vi "Update Trajectory.vi"(5 "Current Surgical Stage":T1(ring), 7 "Pattern":T2(ring)=enum."Centered", 8 "Depth Ctrl Array\n(% Thickness)":dbl[](array[numeric])=[40.0, 60.0, 80.0] min=10.0 max=90.0 step=5.0 format="%#_g%%", 9 "Scale":dbl=0.5, 10 "Offset":dbl[](array[numeric]), 11 "SCAN_NO":string="0011") -> (0 "Trajectory OOB":bool)   [LabVIEW 2016]
uses:
  Subsystems/Global Variables.vi
panel:
  in  "joint limits 1":dbl[][](array[numeric])=[[-8.0, 50.0], [-35.0, 35.0], [-5.0, 20.0], [-180.0, 180.0]] format="%#.3g"
  in  "Total Time":dbl=20.0
  in  "joint limits":dbl[][](array[numeric])=[[-68.0, -4.0], [-35.0, 35.0], [0.1, 10.0], [-40.0, 40.0]]
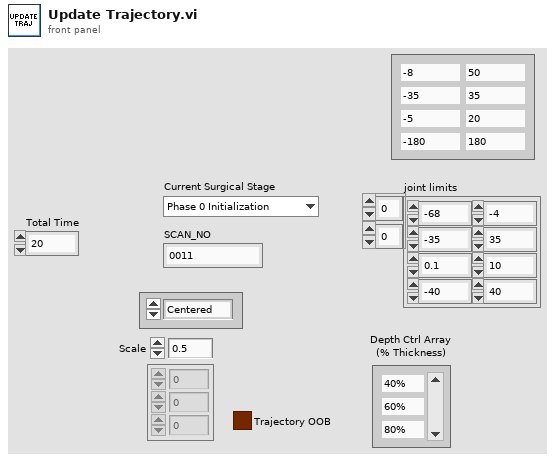
[diagram p1: front panel]
types:
  T1 = enum16{"Phase 0 Initialization", "Phase 1 Phaco", "Phase 2 Lens Removal", "Phase 3 IOL Injection"}
  T2 = enum16{"Entry Site", "Centered", "Insertion", "Extraction", "Reverse Entry Site", "Reverse Centered"}
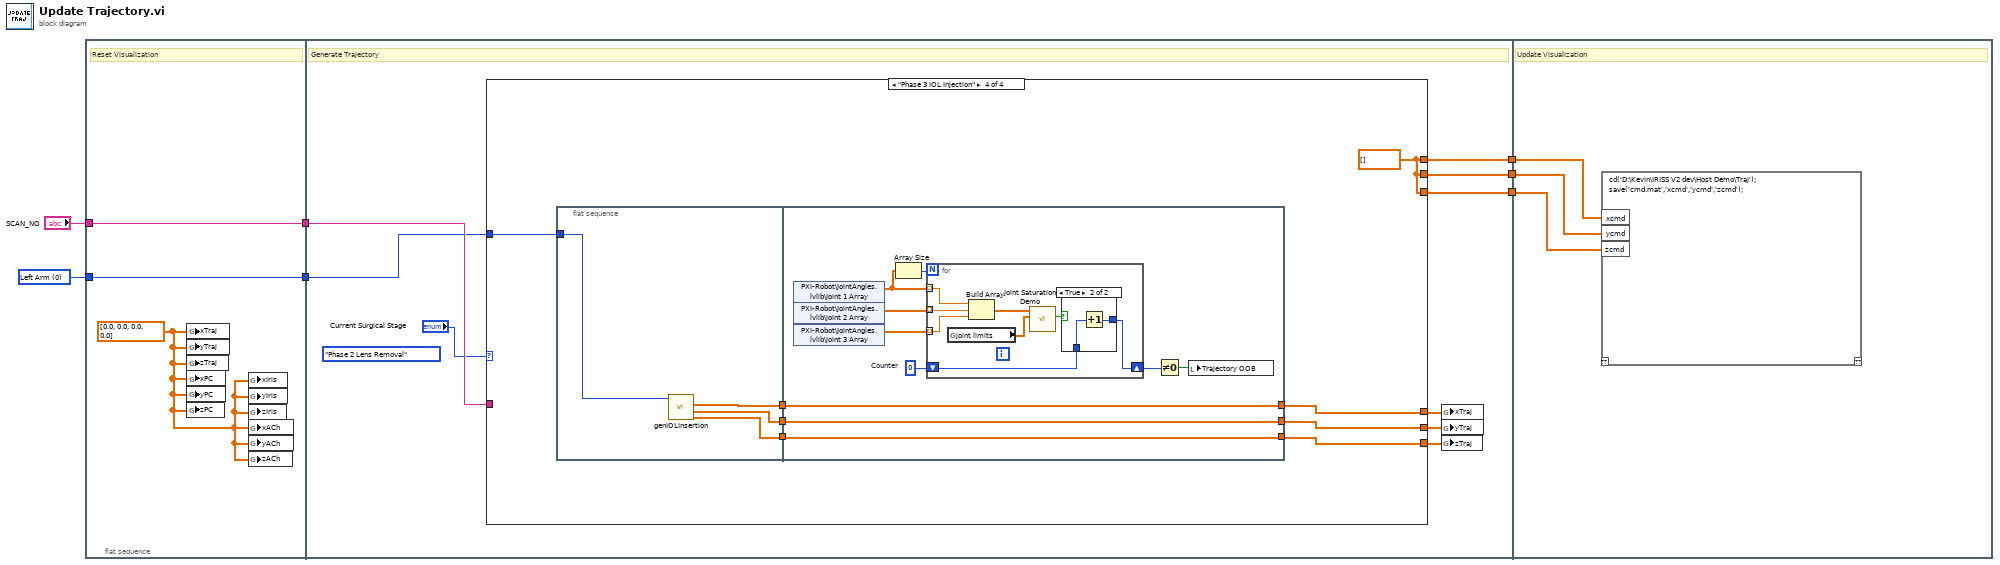
[diagram p0: block diagram]
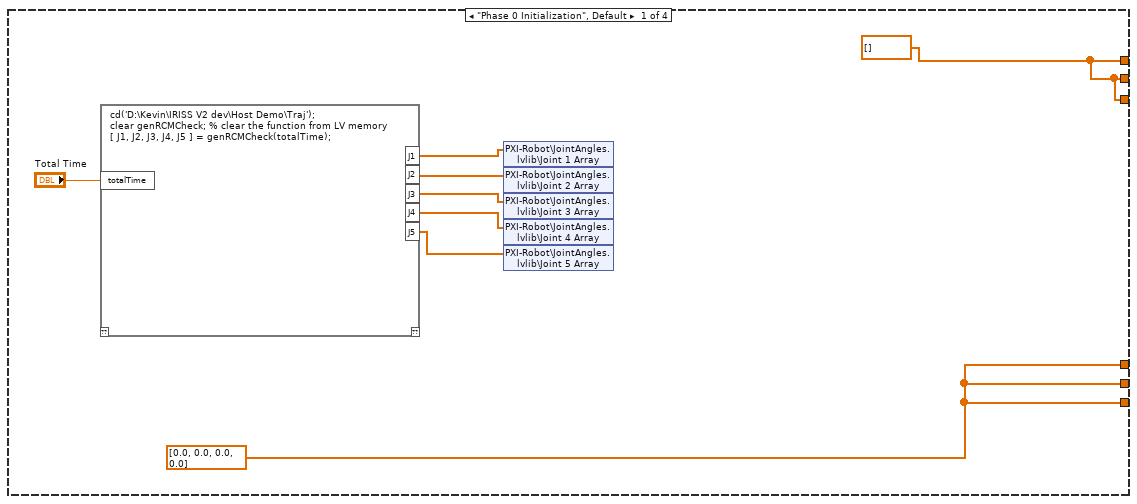
[diagram p2: hidden frame]
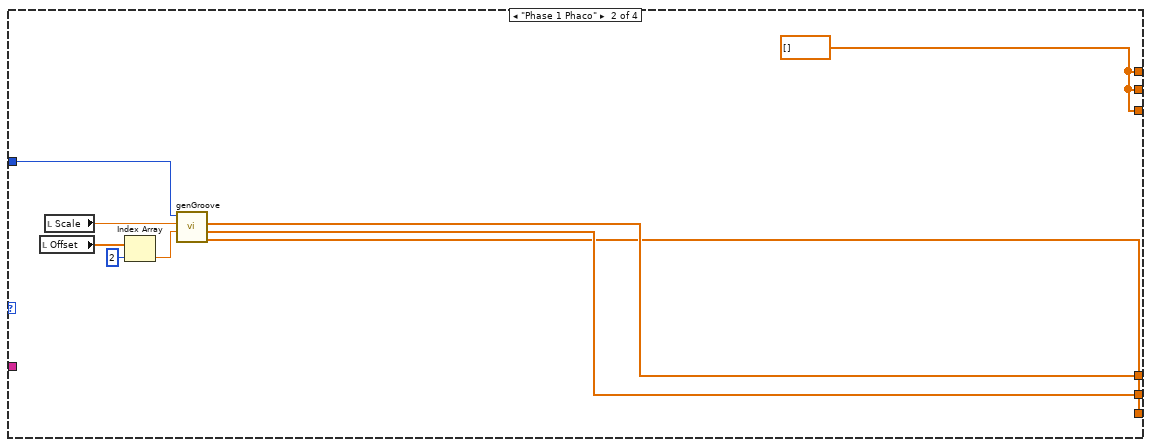
[diagram p3: hidden frame]
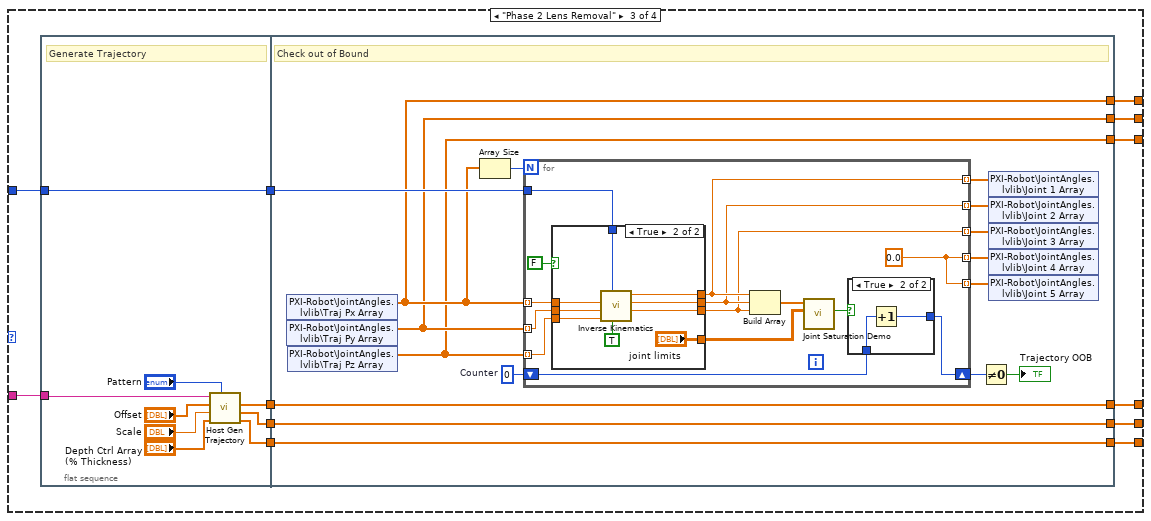
[diagram p4: hidden frame]
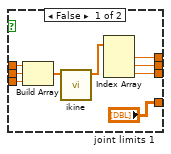
[diagram p5: hidden frame]
diagram:
  w4 = 0 items=["Left Arm", "Right Arm"] ("armID")
  n1 = flat-sequence {
    tunnel: "SCAN_NO" -> [w10]
    tunnel: [w10] -> w7
    tunnel: w4 -> [w8]
    tunnel: [w8] -> w5
    tunnel: w7 -> [w19]
    tunnel: w5 -> [w18]
    tunnel: [w13] -> w3
    tunnel: [w12] -> w2
    tunnel: [w11] -> w1
    tunnel: w3 -> [w144]
    tunnel: w2 -> [w143]
    tunnel: w1 -> [w142]
    frame #0 {
      w9 = dbl[] [0.0, 0.0, 0.0, 0.0] ("First Trk Pt 2")
      # "Reset Visualization"
      n2 = global write "Global Variables.vi" "xTraj"(w9) -> ()
      n3 = global write "Global Variables.vi" "yTraj"(w9) -> ()
      n4 = global write "Global Variables.vi" "zTraj"(w9) -> ()
      n5 = global write "Global Variables.vi" "xPC"(w9) -> ()
      n6 = global write "Global Variables.vi" "yPC"(w9) -> ()
      n7 = global write "Global Variables.vi" "zPC"(w9) -> ()
      n8 = global write "Global Variables.vi" "xIris"(w9) -> ()
      n9 = global write "Global Variables.vi" "yIris"(w9) -> ()
      n10 = global write "Global Variables.vi" "zIris"(w9) -> ()
      n11 = global write "Global Variables.vi" "xACh"(w9) -> ()
      n12 = global write "Global Variables.vi" "yACh"(w9) -> ()
      n13 = global write "Global Variables.vi" "zACh"(w9) -> ()
    }
    frame #1 {
      (unwired) T1."Phase 2 Lens Removal" ("Current Surgical Stage")
      # "Generate Trajectory"
      n14 = case shown="\"Phase 3 IOL Injection\"" "Current Surgical Stage" {
        tunnel: w19 -> [_ _ w48 _]
        tunnel: [w27 w36 w47 w116] -> w17
        tunnel: [w27 w35 w46 w115] -> w16
        tunnel: [w27 w34 w45 w114] -> w15
        tunnel: w18 -> [_ w29 w44 w113]
        tunnel: [w20 w28 w39 w109] -> w13
        tunnel: [w20 w28 w38 w109] -> w12
        tunnel: [w20 w28 w37 w109] -> w11
        frame "Phase 0 Initialization", Default {
          w20 = dbl[] [] ("Array of Double")
          w27 = dbl[] [0.0, 0.0, 0.0, 0.0] ("First Trk Pt 2")
          n15 = script code="cd('D:\\Kevin\\IRISS V2 dev\\Host Demo\\Traj');\nclear genRCMCheck; % clear the function from LV memory\n[ J1, J2, J3, J4, J5 ] = genRCMCheck(totalTime);"("totalTime"="Total Time") -> ("J1"=w25:dbl[], "J2"=w24:dbl[], "J3"=w23:dbl[], "J5"=w21:dbl[], "J4"=w22:dbl[])  [unwired: 1 in, 1 out]
          n16 = shared-variable "PXI-Robot\\JointAngles.lvlib\\Joint 1 Array"(w25) -> ()  [unwired: 1 in, 1 out]
          n17 = shared-variable "PXI-Robot\\JointAngles.lvlib\\Joint 2 Array"(w24) -> ()  [unwired: 1 in, 1 out]
          n18 = shared-variable "PXI-Robot\\JointAngles.lvlib\\Joint 3 Array"(w23) -> ()  [unwired: 1 in, 1 out]
          n19 = shared-variable "PXI-Robot\\JointAngles.lvlib\\Joint 4 Array"(w22) -> ()  [unwired: 1 in, 1 out]
          n20 = shared-variable "PXI-Robot\\JointAngles.lvlib\\Joint 5 Array"(w21) -> ()  [unwired: 1 in, 1 out]
        }
        frame "Phase 1 Phaco" {
          w28 = dbl[] [] ("Array of Double")
          n21 = local read "Offset"() -> (w32:dbl[])
          n22 = local read "Scale"() -> (w33:dbl)
          n23 = Index Array(array=w32, index=2) -> (element=w30:dbl)
          n24 = call "genGroove.vi"("Depth"=w30, "Groove Length"=w33, "armID"=w29) -> ("zVisTraj"=w34:dbl[], "yVisTraj"=w35:dbl[], "xVisTraj"=w36:dbl[])  [unwired: 6 in]
        }
        frame "Phase 2 Lens Removal" {
          n25 = flat-sequence {
            tunnel: w48 -> [w57]
            tunnel: [w56] -> w43
            tunnel: [w55] -> w42
            tunnel: [w54] -> w41
            tunnel: w44 -> [w53]
            tunnel: [w53] -> w40
            tunnel: [w71] -> w45
            tunnel: [w72] -> w46
            tunnel: [w73] -> w47
            tunnel: w43 -> [w73]
            tunnel: w42 -> [w72]
            tunnel: w41 -> [w71]
            tunnel: w40 -> [w70]
            tunnel: [w60] -> w39
            tunnel: [w59] -> w38
            tunnel: [w58] -> w37
            frame #0 {
              # "Generate Trajectory"
              n26 = call "Host Gen Trajectory.vi"("Trajectory Pattern"="Pattern", "Depth Ctrl Array\n(% Thickness)"="Depth Ctrl Array\n(% Thickness)", "Traj Scale Radius from Pupil Radius (Between 0 and 1)"="Scale", "Traj Offset from Pupil Center [mm]"="Offset", "SCAN_NO"=w57) -> ("zVisTraj"=w54:dbl[], "yVisTraj"=w55:dbl[], "xVisTraj"=w56:dbl[])  [unwired: 4 in]
            }
            frame #1 {
              w67 = 0  # Counter
              # "Check out of Bound"
              n27 = shared-variable "PXI-Robot\\JointAngles.lvlib\\Traj Px Array"() -> (w60:dbl[])  [unwired: 1 in, 1 out]
              n28 = shared-variable "PXI-Robot\\JointAngles.lvlib\\Traj Py Array"() -> (w59:dbl[])  [unwired: 1 in, 1 out]
              n29 = shared-variable "PXI-Robot\\JointAngles.lvlib\\Traj Pz Array"() -> (w58:dbl[])  [unwired: 1 in, 1 out]
              n30 = Array Size(array=w60) -> (size(s)=w66:i32)
              n31 = for {
                N: w66 -> [_]
                tunnel: w70 -> [w87]
                tunnel: w60 -> [w86] mode=indexing
                tunnel: w59 -> [w85] mode=indexing
                tunnel: w58 -> [w77] mode=indexing
                shift-right: [w81] -> w68
                shift-left: w67 -> [w82]
                tunnel: [w80] -> w65 mode=indexing
                tunnel: [w79] -> w64 mode=indexing
                tunnel: [w76] -> w63 mode=indexing
                tunnel: [w78] -> w62 mode=indexing
                tunnel: [w78] -> w61 mode=indexing
                w78 = 0.0 ("Numeric")
                n32 = case shown="True" FALSE {
                  tunnel: w87 -> [_ w105]
                  tunnel: w86 -> [w96 w104]
                  tunnel: w85 -> [w95 w103]
                  tunnel: w77 -> [w94 w102]
                  tunnel: [w92 w100] -> w80
                  tunnel: [w91 w99] -> w79
                  tunnel: [w90 w98] -> w76
                  tunnel: ["joint limits 1" "joint limits"] -> w74
                  frame False {
                    n33 = Build Array(w96, w95, w94) -> (w93:dbl[])
                    n34 = call "ikine.vi"("Tip XYZ Posit [mm]"=w93) -> ("Joint Posit [deg,deg,mm]"=w89:dbl[])  [unwired: 10 in]
                    n35 = Index Array(array=w89) -> (element #1=w92:dbl, element #2=w91:dbl, element #3=w90:dbl)  [unwired: 3 in]
                  }
                  frame True {
                    n36 = call "Inverse Kinematics.vi"(6:TRUE ("isToolTipInsideEye"), "armID"=w105, "z"=w102, "y"=w103, "x"=w104) -> ("j3"=w98:dbl, "j2"=w99:dbl, "j1"=w100:dbl)  [unwired: 3 in, 1 out]
                  }
                }
                n37 = Build Array(w80, w79, w76) -> (w84:dbl[])
                n38 = call "Joint Saturation Demo.vi"("Joint Bounds [Deg/mm]"=w74, "Ref Array [Deg/mm]"=w84) -> ("Out of Bound?"=w83:bool)  [unwired: 8 in, 1 out]
                n39 = case shown="True" w83 {
                  tunnel: w82 -> [w106 w108]
                  tunnel: [w106 w107] -> w81
                  frame False {
                  }
                  frame True {
                    n40 = Increment(x=w108) -> (x+1=w107:i32)
                  }
                }
              }
              n41 = Not Equal To 0?(x=w68) -> (x != 0?=→"Trajectory OOB":bool)
              n42 = shared-variable "PXI-Robot\\JointAngles.lvlib\\Joint 1 Array"(w65) -> ()  [unwired: 1 in, 1 out]
              n43 = shared-variable "PXI-Robot\\JointAngles.lvlib\\Joint 2 Array"(w64) -> ()  [unwired: 1 in, 1 out]
              n44 = shared-variable "PXI-Robot\\JointAngles.lvlib\\Joint 3 Array"(w63) -> ()  [unwired: 1 in, 1 out]
              n45 = shared-variable "PXI-Robot\\JointAngles.lvlib\\Joint 4 Array"(w61) -> ()  [unwired: 1 in, 1 out]
              n46 = shared-variable "PXI-Robot\\JointAngles.lvlib\\Joint 5 Array"(w62) -> ()  [unwired: 1 in, 1 out]
            }
          }
        }
        frame "Phase 3 IOL Injection" {
          w109 = dbl[] [] ("Array of Double")
          n47 = flat-sequence {
            tunnel: [w120] -> w112
            tunnel: [w118] -> w111
            tunnel: [w119] -> w110
            tunnel: w113 -> [w117]
            tunnel: [w126] -> w116
            tunnel: [w125] -> w115
            tunnel: [w124] -> w114
            tunnel: w112 -> [w126]
            tunnel: w111 -> [w125]
            tunnel: w110 -> [w124]
            frame #0 {
              n48 = call "genIOLInsertion.vi"("Arm ID Ind"=w117) -> ("zVisTraj"=w119:dbl[], "yVisTraj"=w118:dbl[], "xVisTraj"=w120:dbl[])  [unwired: 8 in]
            }
            frame #1 {
              w129 = 0  # Counter
              n49 = shared-variable "PXI-Robot\\JointAngles.lvlib\\Joint 1 Array"() -> (w121:dbl[])  [unwired: 1 in, 1 out]
              n50 = shared-variable "PXI-Robot\\JointAngles.lvlib\\Joint 2 Array"() -> (w123:dbl[])  [unwired: 1 in, 1 out]
              n51 = shared-variable "PXI-Robot\\JointAngles.lvlib\\Joint 3 Array"() -> (w122:dbl[])  [unwired: 1 in, 1 out]
              n52 = Array Size(array=w121) -> (size(s)=w130:i32)
              n53 = for {
                N: w130 -> [_]
                shift-right: [w134] -> w128
                shift-left: w129 -> [w135]
                tunnel: w121 -> [w133] mode=indexing
                tunnel: w123 -> [w132] mode=indexing
                tunnel: w122 -> [w131] mode=indexing
                n54 = global read "Global Variables.vi" "joint limits"() -> (w138:dbl[][])
                n55 = Build Array(w133, w132, w131) -> (w137:dbl[])
                n56 = call "Joint Saturation Demo.vi"("Joint Bounds [Deg/mm]"=w138, "Ref Array [Deg/mm]"=w137) -> ("Out of Bound?"=w136:bool)  [unwired: 8 in, 1 out]
                n57 = case shown="True" w136 {
                  tunnel: w135 -> [w139 w141]
                  tunnel: [w139 w140] -> w134
                  frame False {
                  }
                  frame True {
                    n58 = Increment(x=w141) -> (x+1=w140:i32)
                  }
                }
              }
              n59 = Not Equal To 0?(x=w128) -> (x != 0?=w127:bool)
              n60 = local write "Trajectory OOB"(w127) -> ()
            }
          }
        }
      }
      n61 = global write "Global Variables.vi" "xTraj"(w17) -> ()
      n62 = global write "Global Variables.vi" "yTraj"(w16) -> ()
      n63 = global write "Global Variables.vi" "zTraj"(w15) -> ()
    }
    frame #2 {
      # "Update Visualization"
      n64 = script code="cd('D:\\Kevin\\IRISS V2 dev\\Host Demo\\Traj');\nsave('cmd.mat','xcmd','ycmd','zcmd');"("xcmd"=w144, "ycmd"=w143, "zcmd"=w142) -> ()  [unwired: 1 in, 1 out]
    }
  }
